vi "Get XY from player particle (SubVI).vi"(4 "Center of mass X":dbl, 5 "Image in Pixels (U8)":u8[][](array[numeric]), 6 "Particle bounding rect bottom":dbl, 7 "Particle bounding rect right":dbl, 8 "Particle bounding rect top":dbl, 9 "Particle bounding rect left":dbl) -> (1 "Y coordinate":i32, 2 "X coordinate":i32)   [LabVIEW 2013]
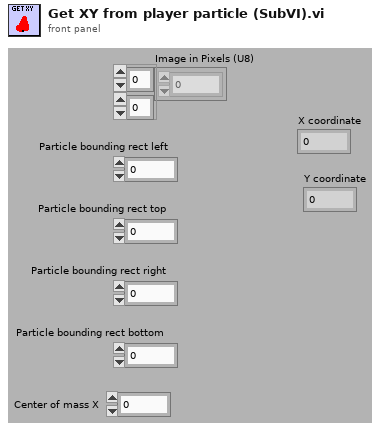
[diagram p1: front panel]
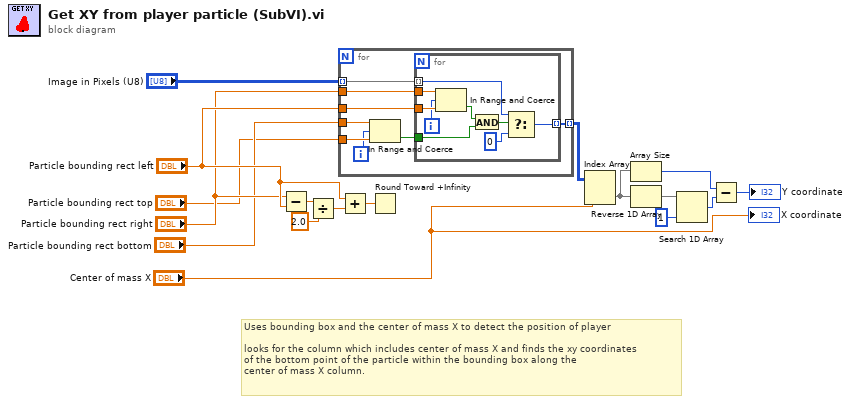
[diagram p0: block diagram]
diagram:
  # "Uses bounding box and the center of mass X to detect the position of player\n\nlooks for the column which includes center of mass X and finds the xy coordinates \nof the bottom point of the particle within the bounding box along the\ncenter of mass X column."
  n1 = Subtract(x="Particle bounding rect right", y="Particle bounding rect left") -> (x-y=w6:dbl)
  n2 = Divide(x=w6, y=2.0) -> (x/y=w9:dbl)
  n3 = for {
    tunnel: "Image in Pixels (U8)" -> [w25] mode=indexing
    tunnel: "Particle bounding rect left" -> [w24]
    tunnel: "Particle bounding rect right" -> [w23]
    tunnel: "Particle bounding rect bottom" -> [w22]
    tunnel: "Particle bounding rect top" -> [w21]
    tunnel: [w18] -> w10 mode=indexing
    i -> [w20]
    n4 = In Range and Coerce(upper limit=w22, x=w20, lower limit=w21) -> (In Range?=w19:bool)  [unwired: 1 out]
    n5 = for {
      tunnel: w25 -> [w26] mode=indexing
      tunnel: w24 -> [w34]
      tunnel: w23 -> [w33]
      tunnel: w19 -> [w32]
      tunnel: [w28] -> w18 mode=indexing
      i -> [w27]
      n6 = In Range and Coerce(upper limit=w33, x=w27, lower limit=w34) -> (In Range?=w31:bool)  [unwired: 1 out]
      n7 = And(x=w31, y=w32) -> (x .and. y?=w30:bool)
      n8 = Select(t=w26, s=w30, f=u8 0) -> (s? t:f=w28:u8)
    }
  }
  n9 = Add(x="Particle bounding rect left", y=w9) -> (x+y=w11:dbl)
  n10 = Round Toward +Infinity(x=w11) -> ()  [unwired: 1 out]
  n11 = Index Array(array=w10, index (col)="Center of mass X") -> (element=w12:u8[])  [unwired: 1 in]
  n12 = Array Size(array=w12) -> (size(s)=w15:i32)
  n13 = Reverse 1D Array(array=w12) -> (reversed array=w13:u8[])
  n14 = Search 1D Array(1D array=w13, element=u8 1) -> (index of element=w16:i32)  [unwired: 1 in]
  n15 = Subtract(x=w15, y=w16) -> (x-y=→"Y coordinate":i32)
  "X coordinate" <- "Center of mass X"
